vi "nominal rid list begin.vi"(8 "error in (no error)":errorcluster, 11 "out_list":i32) -> (0 "error out":errorcluster, 2 "function return":i32, 3 "out_list out":i32)   [LabVIEW 2020, in "client.lvlib"]
doc: "int32_t nominal_rid_list_begin(int32_t *out_list);"
uses:
  client.lvlib
  bin/nominalClient_64.dll
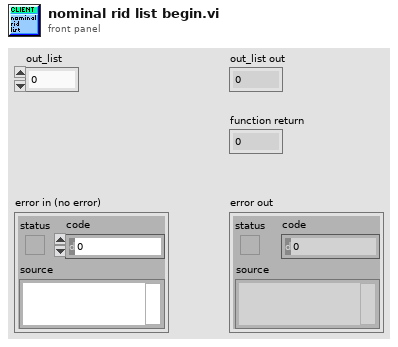
[diagram p1: front panel]
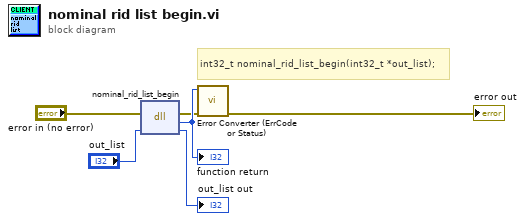
[diagram p0: block diagram]
diagram:
  # "int32_t nominal_rid_list_begin(int32_t *out_list);"
  n1 = dll-call lib="C:/code/labview-client-rs/lv_src/bin/nominalClient_*.*" fn="nominal_rid_list_begin"(error in="error in (no error)", "out_list"="out_list") -> (error out=w2:errorcluster, w6:i32, "out_list"=→"out_list out":i32)  [unwired: 2 in, 1 out]
  "function return" <- w6
  n2 = call "Error Converter (ErrCode or Status).vi"("error in (no error)"=w2, "error code"=w6) -> ("error out"=→"error out":errorcluster)  [unwired: 9 in]
